vi "TrajClosePtAve.vi"(8 "Dmin_Prev":dbl, 9 "ClosePtIdx_Prev":i32, 10 "ClosePtIdx_Target":i32, 11 "TrajLength":i32) -> (1 "weightPrev":dbl, 3 "ClosePtIdx_Ave":i32)   [LabVIEW 2015, in "ForceField.lvclass"]
uses:
  ForceField.lvclass
panel:
  in  "HalfCoeff":dbl=0.05
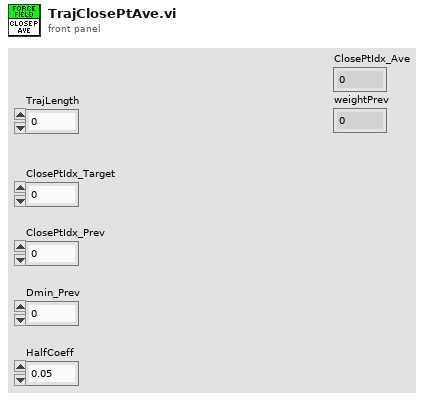
[diagram p1: front panel]
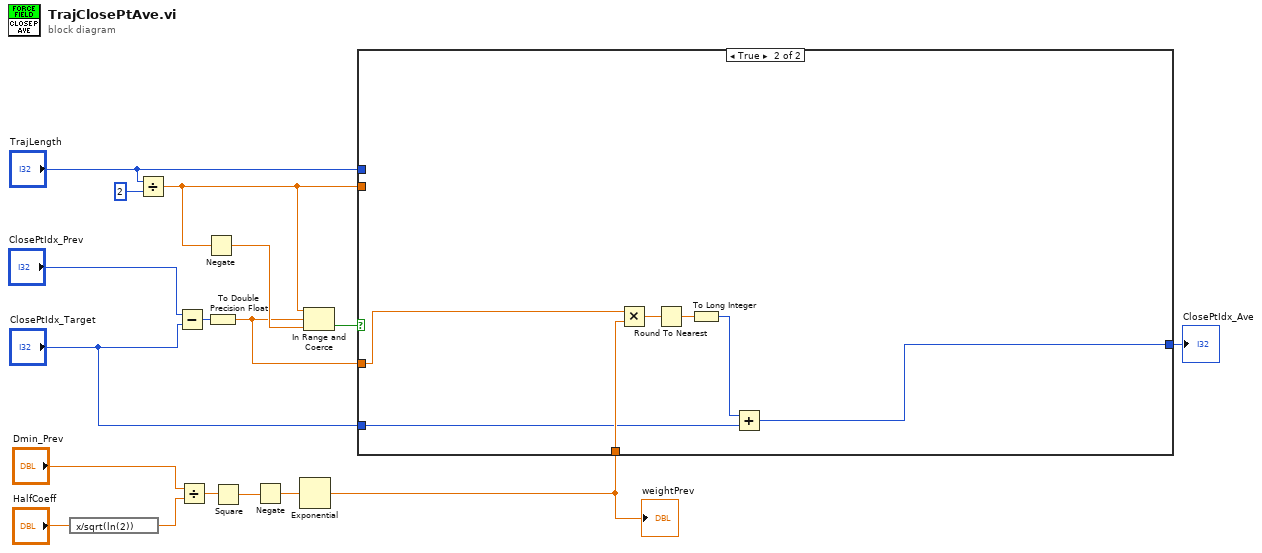
[diagram p0: block diagram]
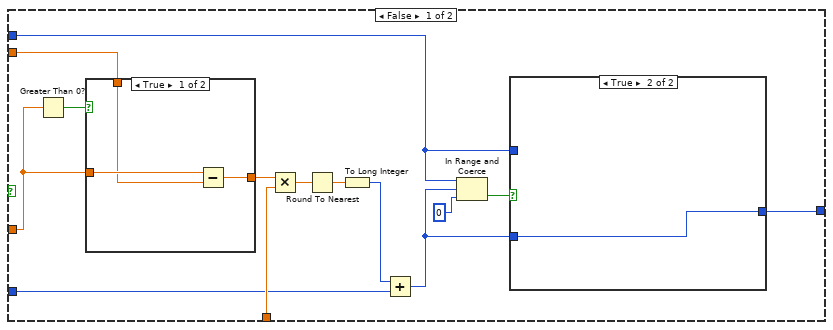
[diagram p2: hidden frame]
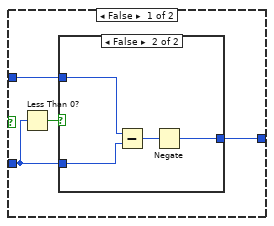
[diagram p3: hidden frame]
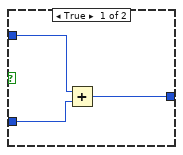
[diagram p4: hidden frame]
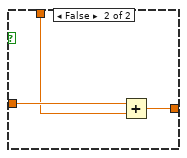
[diagram p5: hidden frame]
diagram:
  n1 = expression code="x/sqrt(ln(2))"("HalfCoeff") -> (w15:dbl)
  n2 = Divide(x="TrajLength", y=2) -> (x/y=w4:dbl)
  n3 = Subtract(x="ClosePtIdx_Prev", y="ClosePtIdx_Target") -> (x-y=w9:i32)
  n4 = Divide(x="Dmin_Prev", y=w15) -> (x/y=w14:dbl)
  n5 = Negate(x=w4) -> (-x=w8:dbl)
  n6 = To Double Precision Float(number=w9) -> (double precision float=w5:dbl)
  n7 = Square(x=w14) -> (x^2=w13:dbl)
  n8 = Negate(x=w13) -> (-x=w12:dbl)
  n9 = Exponential(1:w12) -> (0:w6:dbl)
  "weightPrev" <- w6
  n10 = In Range and Coerce(upper limit=w4, x=w5, lower limit=w8) -> (In Range?=w7:bool)  [unwired: 1 out]
  n11 = case shown="True" w7 {
    tunnel: w6 -> [w27 w56]
    tunnel: w5 -> [w29 w51]
    tunnel: w4 -> [w30 _]
    tunnel: "ClosePtIdx_Target" -> [w26 w55]
    tunnel: "TrajLength" -> [w19 _]
    tunnel: [w18 w50] -> w1
    frame False {
      n12 = Greater Than 0?(x=w29) -> (x > 0?=w31:bool)
      n13 = case shown="True" w31 {
        tunnel: w30 -> [w45 w48]
        tunnel: w29 -> [w46 w49]
        tunnel: [w44 w47] -> w28
        frame True {
          n14 = Subtract(x=w46, y=w45) -> (x-y=w44:dbl)
        }
        frame False {
          n15 = Add(x=w49, y=w48) -> (x+y=w47:dbl)
        }
      }
      n16 = Multiply(x=w28, y=w27) -> (x*y=w25:dbl)
      n17 = Round To Nearest(number=w25) -> (nearest integer value=w24:dbl)
      n18 = To Long Integer(number=w24) -> (32bit integer=w23:i32)
      n19 = Add(x=w23, y=w26) -> (x+y=w20:i32)
      n20 = In Range and Coerce(upper limit=w19, x=w20, lower limit=0) -> (In Range?=w21:bool)  [unwired: 1 out]
      n21 = case shown="True" w21 {
        tunnel: w20 -> [w34 w43]
        tunnel: w19 -> [w33 _]
        tunnel: [w32 w43] -> w18
        frame False {
          n22 = Less Than 0?(x=w34) -> (x < 0?=w35:bool)
          n23 = case shown="False" w35 {
            tunnel: w34 -> [w38 w42]
            tunnel: w33 -> [w37 w41]
            tunnel: [w36 w39] -> w32
            frame True {
              n24 = Add(x=w37, y=w38) -> (x+y=w36:i32)
            }
            frame False {
              n25 = Subtract(x=w41, y=w42) -> (x-y=w40:i32)
              n26 = Negate(x=w40) -> (-x=w39:i32)
            }
          }
        }
        frame True {
        }
      }
    }
    frame True {
      n27 = Multiply(x=w51, y=w56) -> (x*y=w54:dbl)
      n28 = Round To Nearest(number=w54) -> (nearest integer value=w53:dbl)
      n29 = To Long Integer(number=w53) -> (32bit integer=w52:i32)
      n30 = Add(x=w52, y=w55) -> (x+y=w50:i32)
    }
  }
  "ClosePtIdx_Ave" <- w1
